vi "Append text to list.vi"(8 "Text":string, 9 "Up":i32, 10 "Left":i32, 11 "List Text[]":string[][](array[string])) -> (3 "List out[]":string[][](array[string]))   [LabVIEW 2017, in "Popup.lvclass"]
uses:
  Popup.lvclass
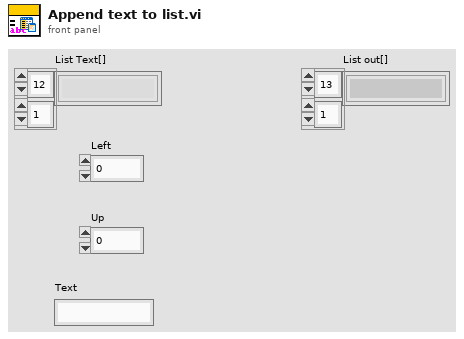
[diagram p1: front panel]
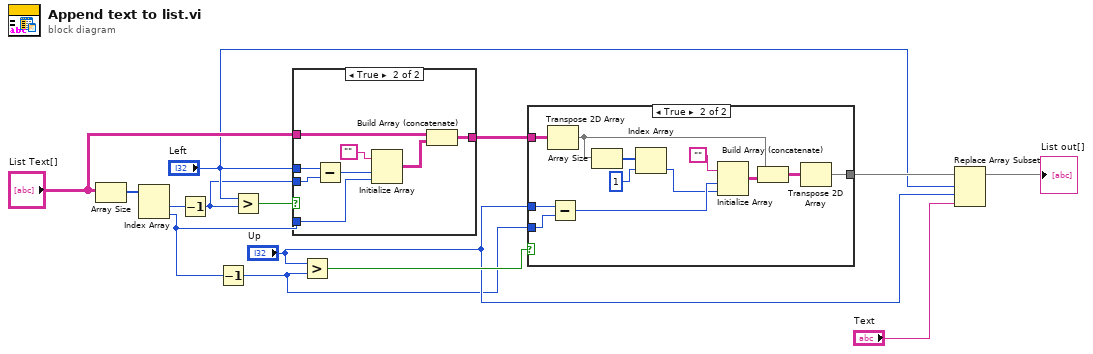
[diagram p0: block diagram]
diagram:
  n1 = Array Size(array="List Text[]") -> (size(s)=w14:i32[])
  n2 = Index Array(array=w14) -> (element #1=w12:i32, element #2=w1:i32)  [unwired: 2 in]
  n3 = Decrement(x=w12) -> (x-1=w3:i32)
  n4 = Decrement(x=w1) -> (x-1=w2:i32)
  n5 = Greater?(x="Left", y=w3) -> (0:w13:bool)
  n6 = case shown="True" w13 {
    tunnel: "Left" -> [_ w23]
    tunnel: w3 -> [_ w22]
    tunnel: "List Text[]" -> [w15 w21]
    tunnel: [w15 w20] -> w10
    tunnel: w1 -> [_ w17]
    frame False {
    }
    frame True {
      n7 = Subtract(x=w23, y=w22) -> (x-y=w19:i32)
      n8 = Initialize Array("", w19, w17) -> (w16:string[][])
      n9 = Build Array (concatenate)(w21, w16) -> (w20:string[][])
    }
  }
  n10 = Greater?(x="Up", y=w2) -> (0:w9:bool)
  n11 = case shown="True" w9 {
    tunnel: "Up" -> [_ w36]
    tunnel: w2 -> [_ w35]
    tunnel: w10 -> [w24 w32]
    tunnel: [w24 w29] -> w8
    frame False {
    }
    frame True {
      n12 = Transpose 2D Array(2D array=w32) -> (transposed array=w28:string[][])
      n13 = Subtract(x=w36, y=w35) -> (x-y=w34:i32)
      n14 = Array Size(array=w28) -> (size(s)=w27:i32[])
      n15 = Index Array(array=w27, index=1) -> (element=w25:i32)
      n16 = Initialize Array("", w34, w25) -> (w31:string[][])
      n17 = Build Array (concatenate)(w28, w31) -> (w30:string[][])
      n18 = Transpose 2D Array(2D array=w30) -> (transposed array=w29:string[][])
    }
  }
  n19 = Replace Array Subset(array=w8, new element="Text", index (row)="Left", index (col)="Up") -> (→"List out[]":string[][])
